vi "Initialise.vi"(8 "error in (no error)":errorcluster, 11 "Queue Sink in":refnum<class "Queue Sink.lvclass">) -> (0 "error out":errorcluster, 3 "Queue Sink out":refnum<class "Queue Sink.lvclass">)   [LabVIEW 2020, in "LV Log.lvlib" / "Queue Sink.lvclass"]
uses:
  Queue Sink.lvclass
  Queue Sink.lvclass/Queue Sink.ctl
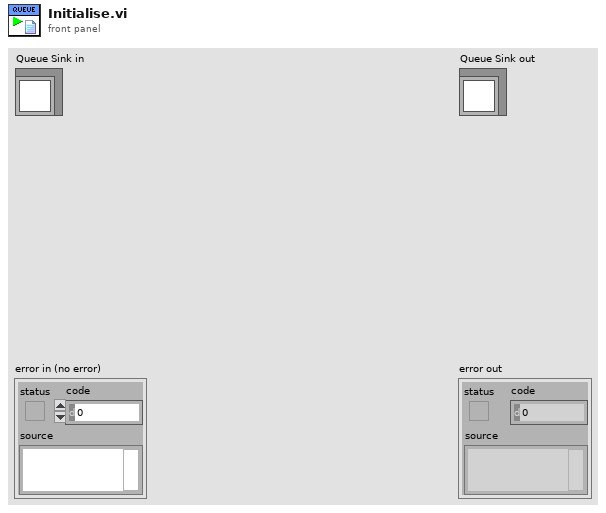
[diagram p1: front panel]
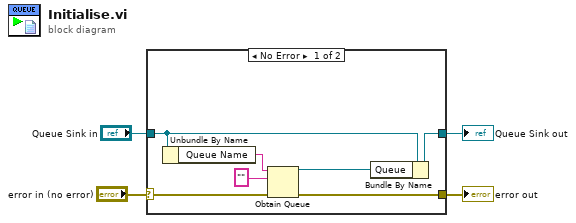
[diagram p0: block diagram]
diagram:
  n1 = case shown="No Error" "error in (no error)" {
    selector: "error in (no error)" -> [w10 w12]
    tunnel: [w9 w12] -> w3
    tunnel: "Queue Sink in" -> [w7 w13]
    tunnel: [w6 w13] -> w1
    frame No Error {
      n2 = Unbundle By Name(w7) -> ("Queue Name"=w8:string)
      n3 = Obtain Queue(name (unnamed)=w8, element data type="", error in (no error)=w10) -> (queue out=w5:refnum<queue>, error out=w9:errorcluster)  [unwired: 2 in, 1 out]
      n4 = Bundle By Name(cluster=w7, "Queue"=w5) -> (w6:refnum<class "Queue Sink.lvclass">)
    }
    frame Error {
    }
  }
  "error out" <- w3
  "Queue Sink out" <- w1
